vi "Actuators Move Absolute Channel.vi"(0 "Notifier Name":string, 2 "Wait to Finish":bool, 5 "Channel":i32, 7 "Position":dbl, 11 "Error In":errorcluster) -> (4 "Notifier Name Out":string, 6 "Channel Out":i32, 15 "Error Out":errorcluster)   [LabVIEW 2025]
uses:
  Actuators Controls/Actuators Note Type.ctl
  Actuators Controls/Actuators Actions.ctl
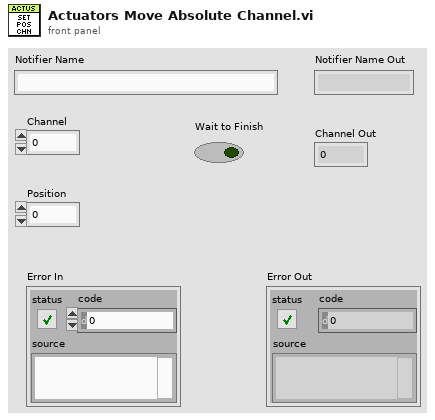
[diagram p1: front panel]
types:
  T1 = typedef "Actuators Note Type.ctl" = cluster{"Actions":T2, "Cmd Received ":bool, "Setpoint":dbl[], "Position":dbl[], "Channel":i32[], "Jog Step":dbl[], "Velocity":dbl[], "Acceleration":dbl[], "Status Bits":u32[], "Moving":bool[]}
  T2 = typedef "Actuators Actions.ctl" = enum16{"Nothing", "Get Position", "Get Acceleration", "Get Velocity", "Get Jog Step", "Set Acceleration", "Set Velocity", "Set Jog Step", "Move Absolute", "Move Relative", "Jog Forward", "Jog Reverse", "Set Moving", "Halt", "Quit"}
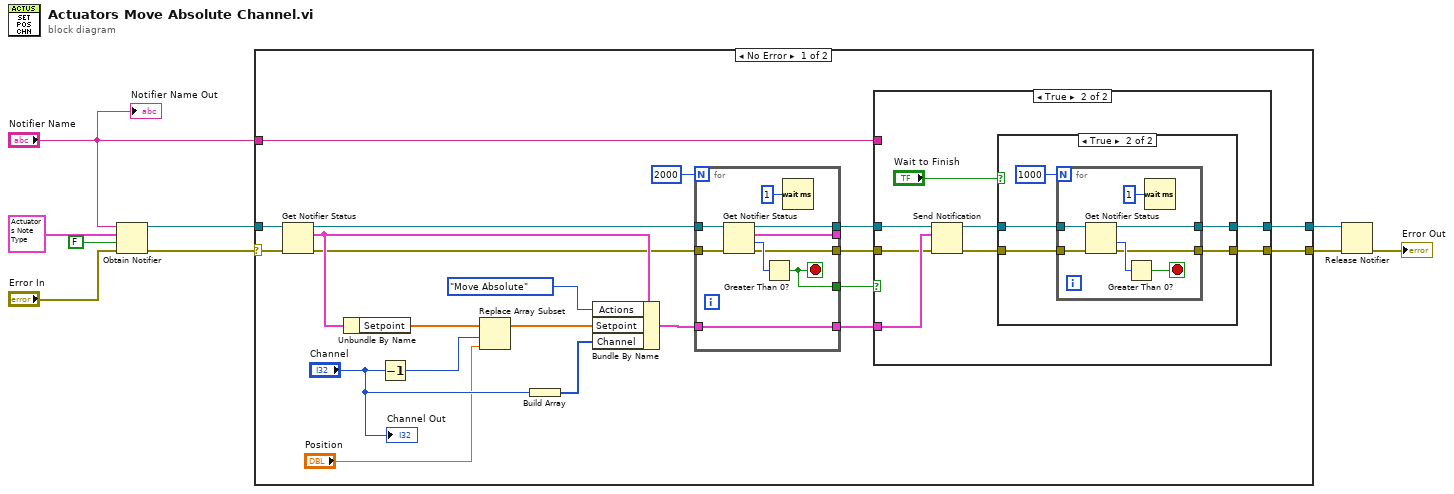
[diagram p0: block diagram]
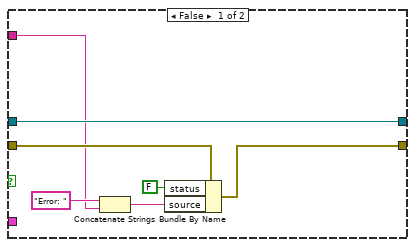
[diagram p2: hidden frame]
diagram:
  n1 = Obtain Notifier(name (unnamed)="Notifier Name", notification data type=T1 {"Actions"=enum."Nothing", "Cmd Received "=FALSE, "Setpoint"=[], "Position"=[], "Channel"=[], "Jog Step"=[], "Velocity"=[], "Acceleration"=[], "Status Bits"=[], "Moving"=[]} ("Actuators Note"), create if not found? (T)=FALSE, error in (no error)="Error In") -> (notifier out=w5:refnum<notifier>, error out=w8:errorcluster)  [unwired: 1 out]
  n2 = case shown="No Error" w8 {
    selector: w8 -> [w23 w69]
    tunnel: w5 -> [w24 w70]
    tunnel: "Notifier Name" -> [w13 _]
    tunnel: [w30 w70] -> w4
    tunnel: [w29 w69] -> w3
    frame No Error {
      n3 = Get Notifier Status(notifier=w24, error in (no error)=w23) -> (notifier out=w20:refnum<notifier>, current notification=w22:T1, error out=w19:errorcluster)  [unwired: 2 out]
      n4 = Unbundle By Name(w22) -> ("Setpoint"=w28:dbl[])
      n5 = Decrement(x="Channel") -> (x-1=w26:i32)
      n6 = Replace Array Subset(array=w28, new element="Position", index=w26) -> (w27:dbl[])
      n7 = Build Array("Channel") -> (w12:i32[])
      n8 = Bundle By Name(cluster=w22, "Actions"=Actuators_Actions."Move Absolute", "Setpoint"=w27, "Channel"=w12) -> (w17:T1)
      n9 = for {
        N: 2000 -> [_]
        tunnel: [w38] -> _
        tunnel: w20 -> [w39]
        tunnel: [w37] -> w15
        tunnel: w19 -> [w34]
        tunnel: [w33] -> w18
        tunnel: [w32] -> w14
        tunnel: w17 -> [w31]
        tunnel: [w31] -> w16
        stop <- w33 stop-if-true
        n10 = Get Notifier Status(notifier=w39, error in (no error)=w34) -> (notifier out=w37:refnum<notifier>, current notification=w38:T1, # waiting=w36:i32, error out=w32:errorcluster)  [unwired: 1 out]
        n11 = Greater Than 0?(x=w36) -> (x > 0?=w33:bool)
        n12 = Wait (ms)(milliseconds to wait=u32 1) -> ()  [unwired: 1 out]
      }
      n13 = case shown="True" w18 {
        tunnel: [w43 w54] -> w30
        tunnel: [w40 w53] -> w29
        tunnel: w16 -> [_ w49]
        tunnel: w15 -> [w43 w48]
        tunnel: w14 -> [w42 w47]
        tunnel: w13 -> [w41 _]
        frame False {
          n14 = Concatenate Strings("Error: " ("source"), w41) -> (w46:string)
          n15 = Bundle By Name(cluster=w42, "status"=FALSE, "source"=w46) -> (w40:errorcluster)
        }
        frame True {
          n16 = Send Notification(notification=w49, notifier=w48, error in (no error)=w47) -> (notifier out=w52:refnum<notifier>, error out=w51:errorcluster)
          n17 = case shown="True" "Wait to Finish" {
            tunnel: w52 -> [w56 w60]
            tunnel: w51 -> [w55 w59]
            tunnel: [w55 w58] -> w53
            tunnel: [w56 w57] -> w54
            frame False {
            }
            frame True {
              n18 = for {
                N: 1000 -> [_]
                tunnel: w60 -> [w68]
                tunnel: [w67] -> w57
                tunnel: w59 -> [w64]
                tunnel: [w62] -> w58
                stop <- w63 stop-if-true
                n19 = Get Notifier Status(notifier=w68, error in (no error)=w64) -> (notifier out=w67:refnum<notifier>, # waiting=w66:i32, error out=w62:errorcluster)  [unwired: 2 out]
                n20 = Greater Than 0?(x=w66) -> (x > 0?=w63:bool)
                n21 = Wait (ms)(milliseconds to wait=u32 1) -> ()  [unwired: 1 out]
              }
            }
          }
        }
      }
      "Channel Out" <- "Channel"
    }
    frame Error {
    }
  }
  n22 = Release Notifier(notifier=w4, error in (no error)=w3) -> (error out=→"Error Out":errorcluster)  [unwired: 1 in, 2 out]
  "Notifier Name Out" <- "Notifier Name"
